vi "InterpolateTemperature.vi"(8 "error in (no error)":errorcluster, 10 "Interpolate Temperature":bool, 11 "Temperature Array In":dbl[](array[numeric])) -> (0 "error out":errorcluster, 3 "Temperature Array Out":dbl[](array[numeric]))   [LabVIEW 2013]
doc: "Use this template to build a VI to use as a subVI."
panel:
  out "XY Graph":cluster{i32[], "Temperature Array In":dbl[]}[](graph)
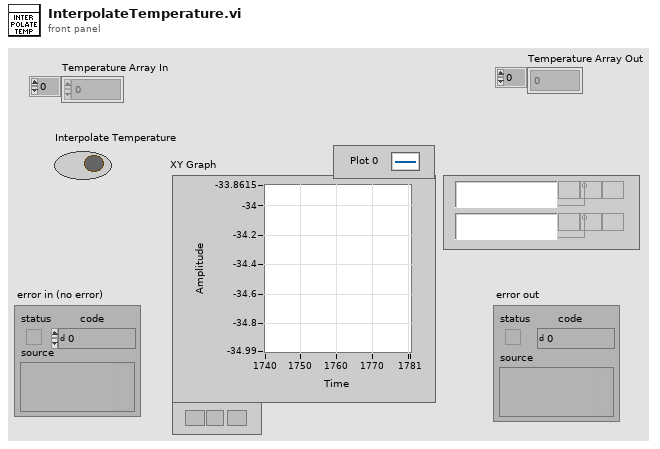
[diagram p1: front panel]
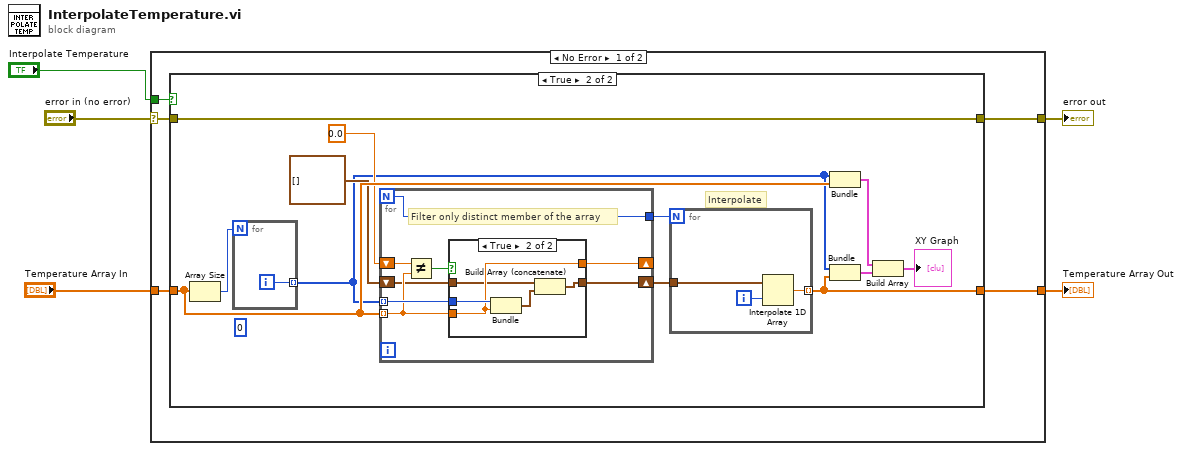
[diagram p0: block diagram]
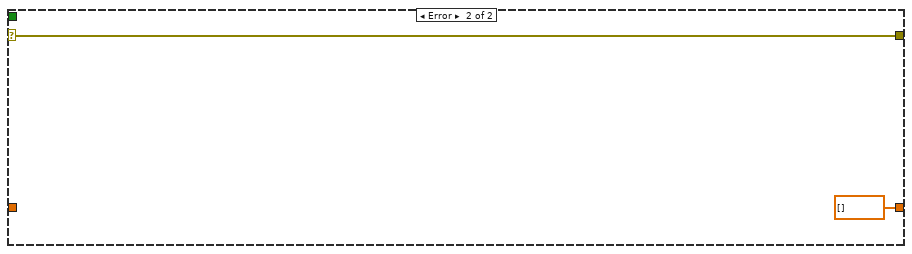
[diagram p4: hidden frame]
diagram:
  n1 = case shown="No Error" "error in (no error)" {
    selector: "error in (no error)" -> [w9 w45]
    tunnel: [w8 w45] -> w4
    tunnel: "Interpolate Temperature" -> [w10 _]
    tunnel: [w7 dbl[] [] ("Temperature Array In")] -> w2
    tunnel: "Temperature Array In" -> [w6 _]
    frame No Error {
      n2 = case shown="True" w10 {
        tunnel: w9 -> [w11 w24]
        tunnel: [w11 w24] -> w8
        tunnel: [w12 w15] -> w7
        tunnel: w6 -> [w12 w22]
        frame False {
        }
        frame True {
          (unwired) 0 ("index")
          # "Interpolate"
          n3 = Array Size(array=w22) -> (size(s)=w23:i32)
          n4 = for {
            N: w23 -> [_]
            tunnel: [w43] -> w16 mode=indexing
            i -> [w43]
          }
          n5 = for {
            N -> [w28]
            tunnel: w16 -> [w33] mode=indexing
            tunnel: w22 -> [w32] mode=indexing
            shift-right: [w30] -> _
            shift-left: 0.0 -> [w35]
            shift-right: [w31] -> w18
            shift-left: cluster{i32, dbl}[] [] -> [w29]
            tunnel: [w28] -> w19
            # "Filter only distinct member of the array"
            n6 = Not Equal?(x=w35, y=w32) -> (x != y?=w34:bool)
            n7 = case shown="True" w34 {
              tunnel: w33 -> [_ w42]
              tunnel: w32 -> [w37 w39]
              tunnel: [w36 w40] -> w31
              tunnel: [w37 w39] -> w30
              tunnel: w29 -> [w36 w38]
              frame False {
              }
              frame True {
                n8 = Bundle(w42, w39) -> (w41:cluster{i32, dbl})  [unwired: 1 in]
                n9 = Build Array (concatenate)(w38, w41) -> (w40:cluster{i32, dbl}[])
              }
            }
          }
          n10 = for {
            N: w19 -> [_]
            tunnel: w18 -> [w27]
            tunnel: [w25] -> w15 mode=indexing
            i -> [w26]
            n11 = Interpolate 1D Array(1:w26, 2:w27) -> (0:w25:dbl)
          }
          n12 = Bundle(w16, "Temperature Array In"=w22) -> (w17:cluster{i32[], "Temperature Array In":dbl[]})  [unwired: 1 in]
          n13 = Bundle(w16, w15) -> (w14:cluster{i32[], dbl[]})  [unwired: 1 in]
          n14 = Build Array(w17, w14) -> (→"XY Graph":cluster{i32[], "Temperature Array In":dbl[]}[])
        }
      }
    }
    frame Error {
    }
  }
  "error out" <- w4
  "Temperature Array Out" <- w2
